vi "HVOF_DAQ.vi"() -> ()   [LabVIEW 2018]
uses:
  <vilib>/Enthought/Python Integration Toolkit/api/Console Visibility.ctl
  Global Variables.vi
  <vilib>/Enthought/Python Integration Toolkit/api/Unpack Double Array.vi
  <vilib>/Enthought/Python Integration Toolkit/Python Integration Toolkit.lvlib
  <vilib>/Analysis/NI_AALPro.lvlib
panel:
  in  "Clear":bool
  out "Delta T (water)":cluster{"X":dbl[], "Y":dbl[]}(graph)={"X"=[3626976328.9747047, 3626976329.2882648, 3626976329.537915, 3626976329.7875648, 3626976330.037215, 3626976330.2868648, 3626976330.536515, 3626976330.7861648, 3626976331.0358152, 3626976331.2844663, 3626976331.5341167, 3626976331.7837663, 3626976332.0334167, 3626976332.2830663, 3626976332.5327168, 3626976332.7823663, 3626976333.0320168, 3626976333.2816663, 3626976333.5313168, 3626976333.7809663, 3626976334.0306168, 3626976334.2802663, 3626976334.529917, 3626976334.7795663, 3626976335.029217, 3626976335.2788663, 3626976335.528517, 3626976335.7781663, 3626976336.027817, 3626976336.2774663, 3626976336.527117, 3626976336.7767663, 3626976337.026417, 3626976337.2760663, 3626976337.525717, 3626976337.7753663, 3626976338.025017, 3626976338.2746663, 3626976338.524317, 3626976338.7739663, 3626976339.023617, 3626976339.2732663, 3626976339.522917, 3626976339.7725663, 3626976340.022217, 3626976340.2718663, 3626976340.521517, 3626976340.7711663, 3626976341.020817, 3626976341.2704663, 3626976341.520117, 3626976341.7697663, 3626976342.019417, 3626976342.2690663, 3626976342.518717, 3626976342.7683663, 3626976343.018017, 3626976343.2676663, 3626976343.517317, 3626976343.7669663, 3626976344.016617, 3626976344.2662663, 3626976344.515917, 3626976344.7655663], "Y"=[0.016941995376026142, -0.0034307203438679323, -0.0012931560773346007, 0.010212766094994663, -0.0005542021339124403, -0.0017151365641332461, -0.0034042597751167136, 0.008075112661089179, 0.013062579982253908, -0.0017947808146345778, -0.00029020971273041596, -0.0277087398070357, -0.006043112142130269, 0.005251339553606016, 0.004908344665242481, -0.027207278935801327, -0.018287754627294817, 0.004037512931798659, 0.020003009075523437, 0.001715165849578426, 0.01781288109937762, 0.013511391362559522, -0.0009499695656778329, 0.0052251496198962855, -0.00475004623102393, 0.014091761079061627, 0.004354215535926187, -0.004143001067557606, 0.0008971989165296179, 0.0018736020359426675, 0.015543342306873598, 0.004459598401435727, -0.011294751416421889, 0.004275060252105334, -0.010450252501527757, -0.009605758581823665, 0.008154198125065903, 0.02092663018909846, -0.019185110047445164, -0.015358660324153561, -0.009447532053005858, -0.0005277680540594076, 0.009130734924596595, 0.01063513118945636, -0.00794342524870828, 0.008945990824315686, -0.008154211481919305, -0.00451269963069123, -0.005146015504564616, -0.0009762739930785358, -2.661033007456126e-05, 0.012745861399210412, -0.00044865324857923383, 0.005277504139456823, 0.006491598743970428, 0.004010972658196721, 0.0030610687129772884, -0.00451262343150205, 0.0032459063136975885, 0.0017681774285875917, -0.009763964236483957, -0.005330620501556638, -0.0016362406714414135, 0.027128009392132668]}
  in  "Clear":bool
  out "General XY Graph":cluster{"Y":dbl[], "Y":dbl[]}[](graph)=[{"Y"=[3626976328.9747047, 3626976329.2882648, 3626976329.537915, 3626976329.7875648, 3626976330.037215, 3626976330.2868648, 3626976330.536515, 3626976330.7861648, 3626976331.0358152, 3626976331.2844663, 3626976331.5341167, 3626976331.7837663, 3626976332.0334167, 3626976332.2830663, 3626976332.5327168, 3626976332.7823663, 3626976333.0320168, 3626976333.2816663, 3626976333.5313168, 3626976333.7809663, 3626976334.0306168, 3626976334.2802663, 3626976334.529917, 3626976334.7795663, 3626976335.029217, 3626976335.2788663, 3626976335.528517, 3626976335.7781663, 3626976336.027817, 3626976336.2774663, 3626976336.527117, 3626976336.7767663, 3626976337.026417, 3626976337.2760663, 3626976337.525717, 3626976337.7753663, 3626976338.025017, 3626976338.2746663, 3626976338.524317, 3626976338.7739663, 3626976339.023617, 3626976339.2732663, 3626976339.522917, 3626976339.7725663, 3626976340.022217, 3626976340.2718663, 3626976340.521517, 3626976340.7711663, 3626976341.020817, 3626976341.2704663, 3626976341.520117, 3626976341.7697663, 3626976342.019417, 3626976342.2690663, 3626976342.518717, 3626976342.7683663, 3626976343.018017, 3626976343.2676663, 3626976343.517317, 3626976343.7669663, 3626976344.016617, 3626976344.2662663, 3626976344.515917, 3626976344.7655663], "Y"=[5.746555713603573, 5.699783191946977, 5.753300065910536, 5.739767563942959, 5.784591234930852, 5.742044879207851, 5.834560760793132, 5.76162102278082, 5.800357252816253, 5.787463095545072, 5.768518652631912, 5.719227948241672, 5.777211861182645, 5.701929124682287, 5.720081940981363, 5.754241647220031, 5.742066778961799, 5.737599740402041, 5.763635566989369, 5.7283372027544965, 5.772876208570432, 5.765693913205542, 5.800291565032008, 5.781875977763636, 5.753190579724322, 5.778175339779396, 5.71064422770916, 5.718023598797108, 5.781963568315495, 5.761489637889099, 5.715155056662675, 5.780496451876758, 5.693892828585813, 5.765321656561875, 5.692338130932262, 5.795802625382005, 5.7746936776866535, 5.757570026557633, 5.7393515193935585, 5.791707843718633, 5.7383880394743105, 5.727811667047649, 5.7434244077143, 5.7520081297636265, 5.719030872886687, 5.690849111997867, 5.745679827512527, 5.7247898475659245, 5.755993424890152, 5.74605207668688, 5.724877438603042, 5.756212400427707, 5.7649494023393375, 5.757438645681126, 5.747935241465974, 5.7416069330134265, 5.73922013403042, 5.717016329940236, 5.716118537338039, 5.703067780408296, 5.767993119931336, 5.77541628947981, 5.725271587807375, 5.741278477750302]}]
  in  "Display":T1(ring)
  in  "Clear":bool caption="Reset"
  out "dM/dt (seed)":cluster{"X":dbl[], "Y":dbl[]}(graph)={"X"=[3626976329.2882648, 3626976329.537915, 3626976329.7875648, 3626976330.037215, 3626976330.2868648, 3626976330.536515, 3626976330.7861648, 3626976331.0358152, 3626976331.2844663, 3626976331.5341167, 3626976331.7837663, 3626976332.0334167, 3626976332.2830663, 3626976332.5327168, 3626976332.7823663, 3626976333.0320168, 3626976333.2816663, 3626976333.5313168, 3626976333.7809663, 3626976334.0306168, 3626976334.2802663, 3626976334.529917, 3626976334.7795663, 3626976335.029217, 3626976335.2788663, 3626976335.528517, 3626976335.7781663, 3626976336.027817, 3626976336.2774663, 3626976336.527117, 3626976336.7767663, 3626976337.026417, 3626976337.2760663, 3626976337.525717, 3626976337.7753663, 3626976338.025017, 3626976338.2746663, 3626976338.524317, 3626976338.7739663, 3626976339.023617, 3626976339.2732663, 3626976339.522917, 3626976339.7725663, 3626976340.022217, 3626976340.2718663, 3626976340.521517, 3626976340.7711663, 3626976341.020817, 3626976341.2704663, 3626976341.520117, 3626976341.7697663, 3626976342.019417, 3626976342.2690663, 3626976342.518717, 3626976342.7683663, 3626976343.018017, 3626976343.2676663, 3626976343.517317, 3626976343.7669663, 3626976344.016617, 3626976344.2662663, 3626976344.515917, 3626976344.7655663], "Y"=[-2.5294209395323057e-06, -4.259990571658549e-09, -1.2808149425667877e-11, 1.8085107227541341e-09, -5.379422771258245e-10, 1.5113616308576627e-10, 1.424266238208227e-09, 7.275029040386229e-10, -6.475231197382718e-10, 2.089720763854891e-09, -1.1450485775236743e-09, -1.3013079992401613e-09, 1.8981677703537083e-09, -1.0246515663609178e-11, -3.299379341274009e-09, -4.867097574581571e-11, -2.203001731242689e-09, 2.4950275467482267e-09, -2.3233983482318323e-09, 3.112380365943664e-09, -2.5769997091317265e-09, 3.885992600931171e-09, -1.869989848959745e-09, 2.1210295811829608e-09, -3.6118981658193606e-10, 3.775842497494251e-09, -4.651919934613945e-09, 1.869989846723482e-09, -5.338436771311457e-09, 5.8405162360633124e-09, -6.480923716412123e-09, 4.3522092517814356e-09, -4.651919953105369e-09, 5.520312497129659e-09, -5.507504346244076e-09, 7.257097584244414e-09, -2.23117966599756e-09, 2.664095121156259e-09, -3.276324674057799e-09, 3.873184442553429e-09, -2.5129589512684207e-09, 2.4822193848779224e-09, -5.153999395455975e-09, 1.6727443400957462e-09, -3.4351457380716585e-09, 1.4729372115131607e-09, -3.417214324594375e-09, 3.199475776996257e-09, -2.5949311204870922e-09, 6.2017060580144864e-09, -3.0790791737566973e-09, 3.809143702552645e-09, -2.279850629196931e-09, 4.449551178950508e-09, -4.444427917915515e-09, 4.380387168823738e-09, -5.940419799412757e-09, 4.252305674276681e-09, -2.748628906753415e-09, 4.201073105044614e-10, -2.3438913778313254e-09, 4.4572359918503736e-10, -1.7931409476573773e-09]}
  out "M (seed)":cluster{"X":dbl[], "Y":dbl[]}[](graph)=[{"X"=[3626976328.9747047, 3626976329.2882648, 3626976329.537915, 3626976329.7875648, 3626976330.037215, 3626976330.2868648, 3626976330.536515, 3626976330.7861648, 3626976331.0358152, 3626976331.2844663, 3626976331.5341167, 3626976331.7837663, 3626976332.0334167, 3626976332.2830663, 3626976332.5327168, 3626976332.7823663, 3626976333.0320168, 3626976333.2816663, 3626976333.5313168, 3626976333.7809663, 3626976334.0306168, 3626976334.2802663, 3626976334.529917, 3626976334.7795663, 3626976335.029217, 3626976335.2788663, 3626976335.528517, 3626976335.7781663, 3626976336.027817, 3626976336.2774663, 3626976336.527117, 3626976336.7767663, 3626976337.026417, 3626976337.2760663, 3626976337.525717, 3626976337.7753663, 3626976338.025017, 3626976338.2746663, 3626976338.524317, 3626976338.7739663, 3626976339.023617, 3626976339.2732663, 3626976339.522917, 3626976339.7725663, 3626976340.022217, 3626976340.2718663, 3626976340.521517, 3626976340.7711663, 3626976341.020817, 3626976341.2704663, 3626976341.520117, 3626976341.7697663, 3626976342.019417, 3626976342.2690663, 3626976342.518717, 3626976342.7683663, 3626976343.018017, 3626976343.2676663, 3626976343.517317, 3626976343.7669663, 3626976344.016617, 3626976344.2662663, 3626976344.515917, 3626976344.7655663], "Y"=[-9182.465313225688, -9174.149894063119, -9189.60077906248, -9189.647233917369, -9183.08780832068, -9185.038912230502, -9184.490744943321, -9179.324964999714, -9176.686329181648, -9179.034880214616, -9171.455512453122, -9175.608576548546, -9180.328389868973, -9173.443780282194, -9173.480944152043, -9185.447714949718, -9185.624243427048, -9193.614478576694, -9184.565072704409, -9192.991983534932, -9181.703453595828, -9191.050170561373, -9176.955767351936, -9183.738176284593, -9176.045252183509, -9177.355279101426, -9163.660387710675, -9180.532791235262, -9173.750382310716, -9193.112766156975, -9171.929351972754, -9195.435508934255, -9179.650148964256, -9196.52255255591, -9176.50050975583, -9196.476097695728, -9170.15477648218, -9178.247212334409, -9168.584602370387, -9180.467754435611, -9166.41980611353, -9175.5342487657, -9166.531297793439, -9185.224731641807, -9179.157727502385, -9191.616919808608, -9186.274611396524, -9198.668766890376, -9187.064343956321, -9196.476097726541, -9173.982656604929, -9185.150403907975, -9171.334729834483, -9179.603694118536, -9163.465277282094, -9179.585112171993, -9163.697551563655, -9185.243313608129, -9169.820301549724, -9179.789513553786, -9178.265794279574, -9186.767032843529, -9185.15040389643, -9191.654083682537]}]
  in  "Seed Channel":i32=2
  out "Data":T2={"Fuel Flow\n(L/hr)"=5.741278477750302, "O2 Flow\n(SLPM)"=0.0, "Phi"=-inf, "Q_water "=1.0866120412865794e-05, "Q_fuel"=-2.595149921295117e-10, "Delta T (C)"=0.027128009392132668, "Water Flow\n(L/min)"=5.741278477750302, "Chamber Pressure (PSI)"=14.690853351832978} {"Chamber Pressure (PSI)" scale=0.0..30.0; "Water Flow\n(L/min)" scale=6.0..40.0; "Delta T (C)" scale=0.0..100.0; "O2 Flow\n(SLPM)" scale=0.0..600.0; "Phi" scale=0.0..2.0; "Fuel Flow\n(L/hr)" scale=6.0..16.0; "Q_water" format="%#_3g"; "Q_fuel" format="%#_3g"}
  in  "stop":bool
  # "Torch"
  # "Fuel In"
  # "O2 In"
  # "Water In"
  # "Water Out"
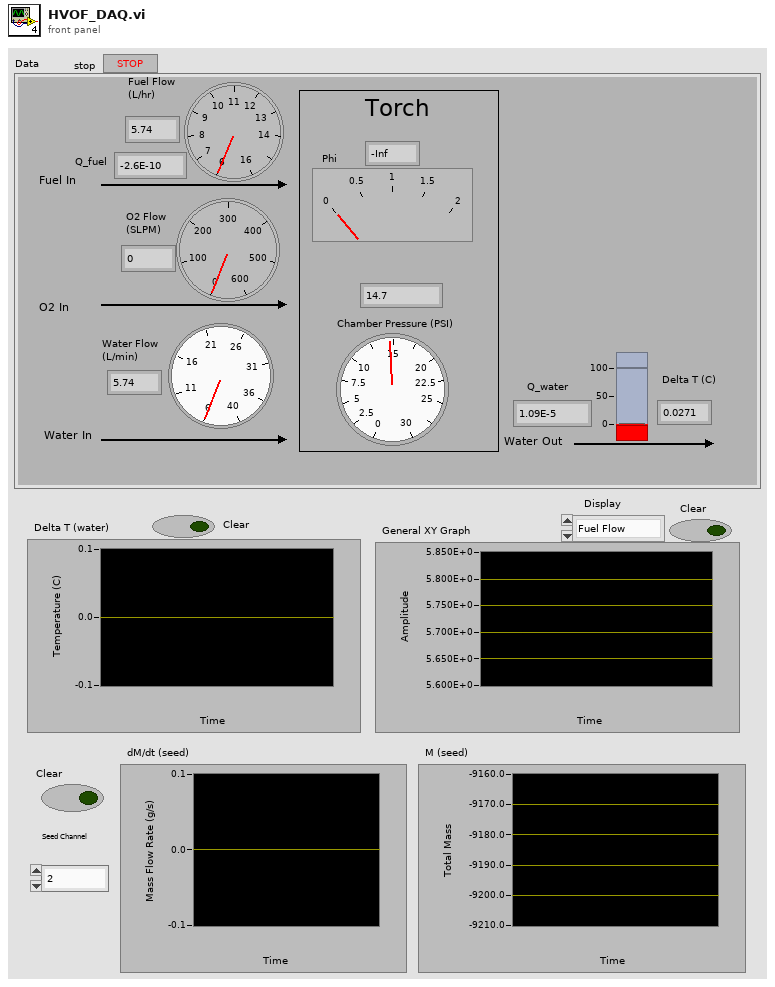
[diagram p1: front panel]
types:
  T1 = enum16{"Fuel Flow", "O2 Flow", "Phi", "Q_water", "Q_Fuel", "Delta T", "Water Flow", "Chamber Pressure"}
  T2 = cluster{"Fuel Flow\n(L/hr)":dbl, "O2 Flow\n(SLPM)":dbl, "Phi":dbl, "Q_water ":dbl, "Q_fuel":dbl, "Delta T (C)":dbl, "Water Flow\n(L/min)":dbl, "Chamber Pressure (PSI)":dbl}
  T3 = typedef "Python Integration Toolkit.lvlib/Console Visibility.ctl" = enum16{"Show Console", "Show Console While Running", "Hide Console"}
  T4 = typedef "Python Integration Toolkit.lvlib/Session ID.ctl" = u64
  T5 = typedef "Python Integration Toolkit.lvlib/Python Objects.ctl" = variant
  T6 = cluster{dbl, dbl, "Numeric":dbl, "Numeric":dbl, "Numeric":dbl, dbl, dbl, dbl}
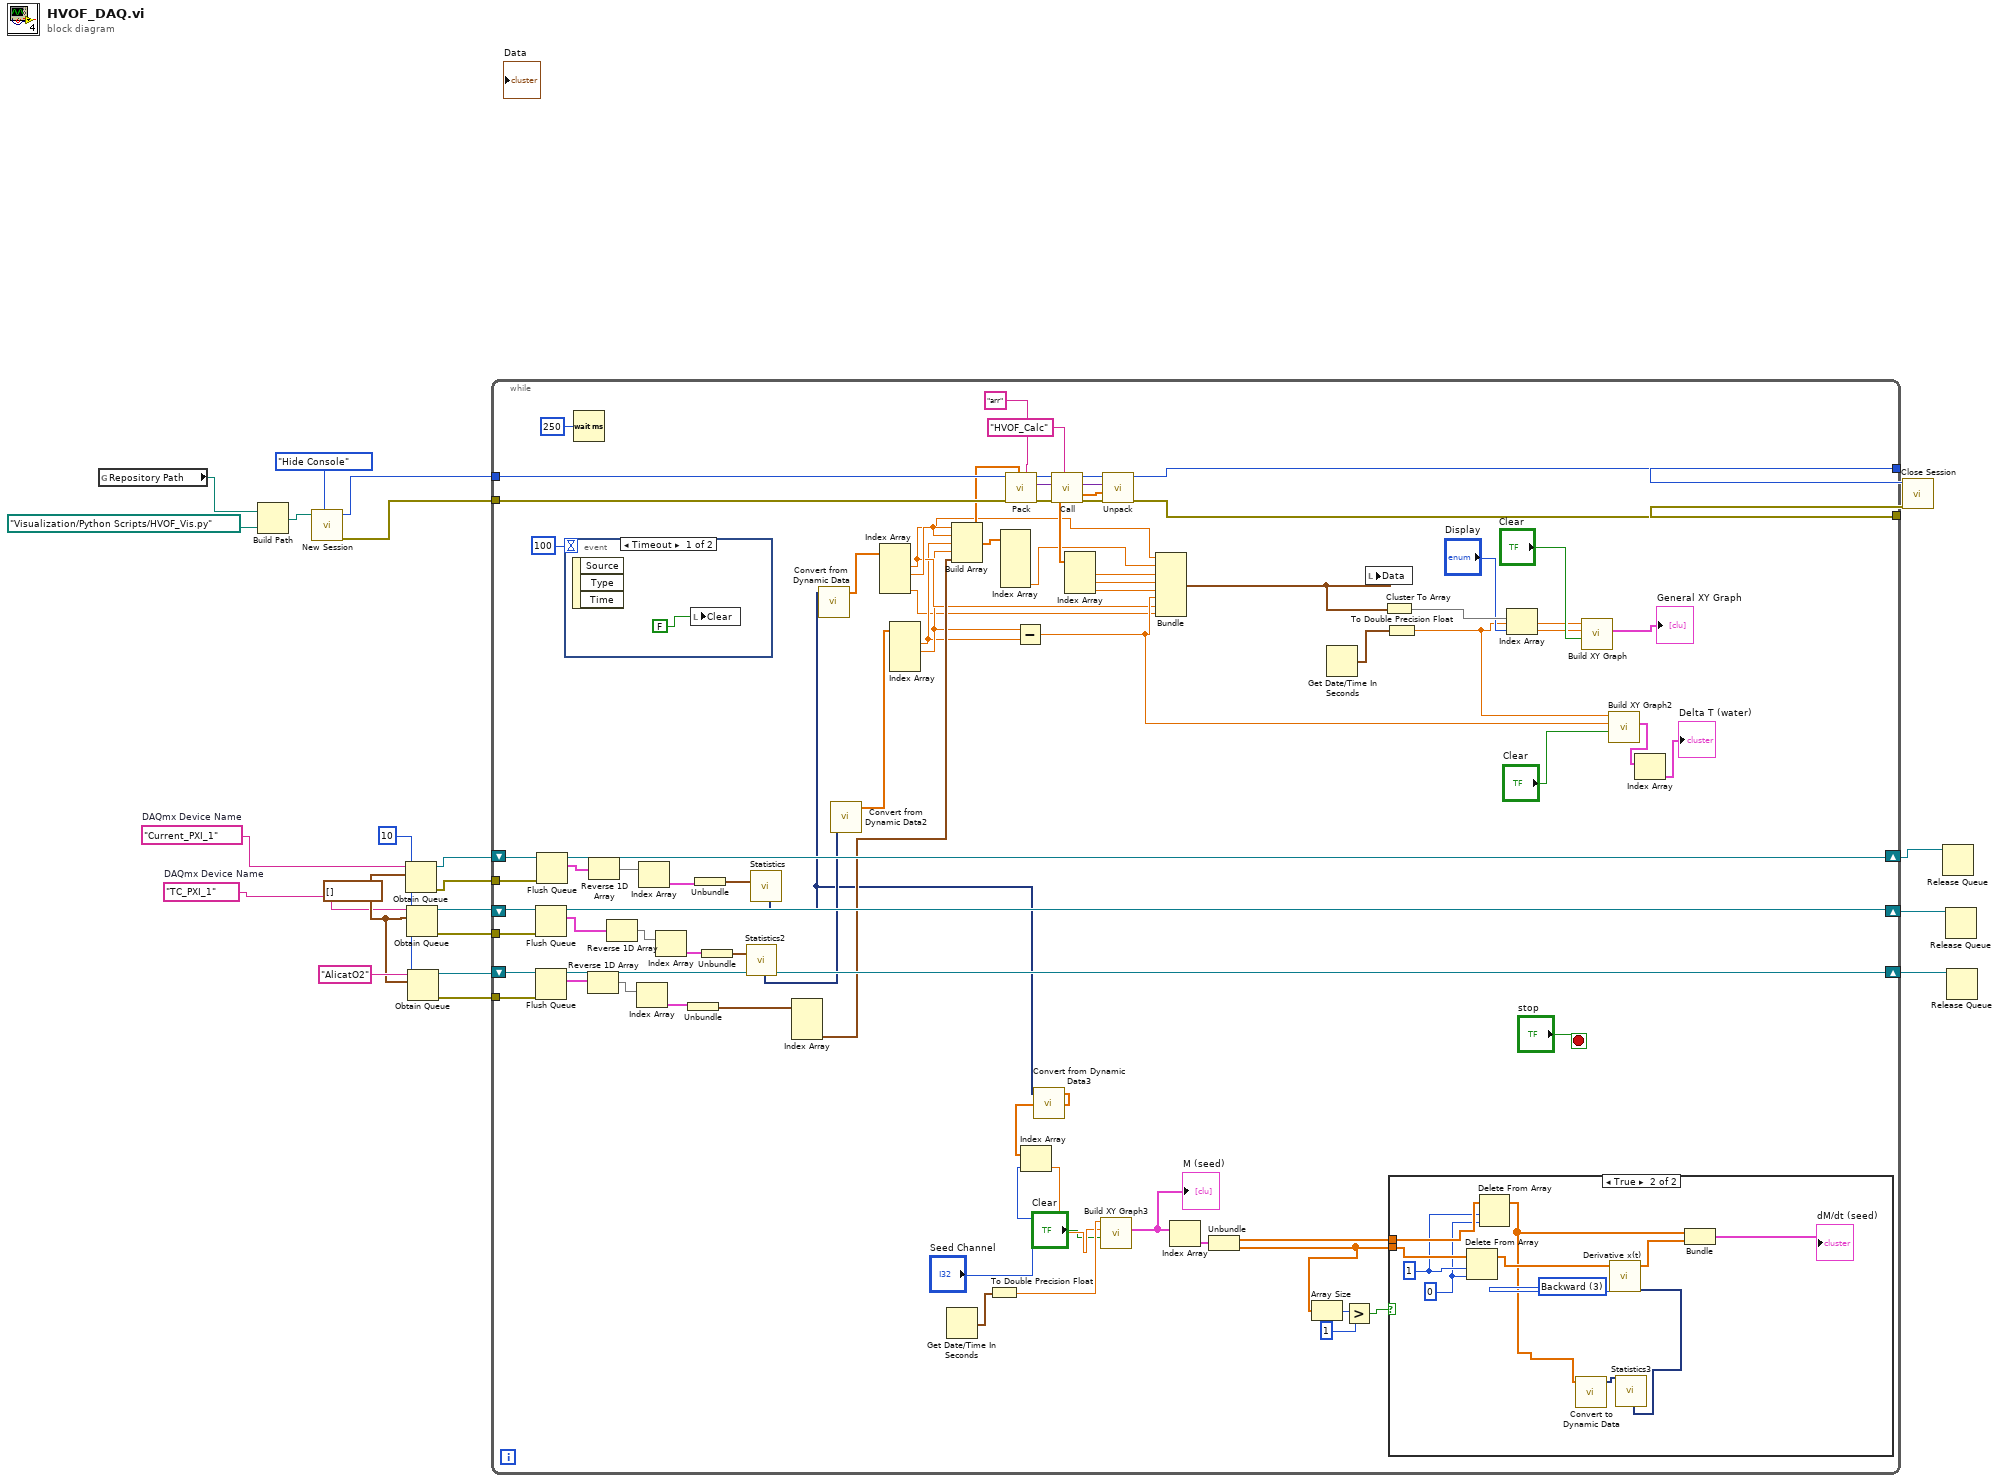
[diagram p0: block diagram]
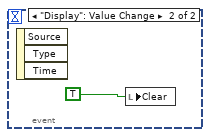
[diagram p3: hidden frame]
diagram:
  w1 = tag "TC_PXI_1"  # DAQmx Device Name
  w2 = tag "Current_PXI_1"  # DAQmx Device Name
  w17 = waveform(dbl)[] [] ("data")
  w6 = 10 ("max queue size (-1, unlimited)")
  n1 = global read "Global Variables.vi" "Repository Path"() -> (w11:path)
  n2 = Build Path(base path=w11, name or relative path=path "Visualization/Python Scripts/HVOF_Vis.py" ("vi path")) -> (appended path=w13:path)
  n3 = call <vilib>:"New Session.vi"("Console Visibility"=Console_Visibility."Hide Console", "Path to Python Module (.py File)"=w13) -> ("error out"=w9:errorcluster, "Session ID out"=w10:T4)  [unwired: 8 in]
  n4 = Obtain Queue(max queue size (-1, unlimited)=w6, name (unnamed)=w2, element data type=w17) -> (queue out=w22:refnum<queue>, error out=w20:errorcluster)  [unwired: 2 in, 1 out]
  n5 = Obtain Queue(max queue size (-1, unlimited)=w6, name (unnamed)=w1, element data type=w17) -> (queue out=w21:refnum<queue>, error out=w19:errorcluster)  [unwired: 2 in, 1 out]
  n6 = Obtain Queue(max queue size (-1, unlimited)=w6, name (unnamed)="AlicatO2", element data type=w17) -> (queue out=w16:refnum<queue>, error out=w15:errorcluster)  [unwired: 2 in, 1 out]
  n7 = while {
    shift-right: [w95] -> w4
    shift-left: w21 -> [w97]
    shift-right: [w96] -> w5
    shift-left: w22 -> [w98]
    tunnel: w20 -> [w92]
    tunnel: w19 -> [w91]
    shift-right: [w80] -> w3
    shift-left: w16 -> [w83]
    tunnel: w15 -> [w79]
    tunnel: w10 -> [w78]
    tunnel: w9 -> [w77]
    tunnel: [w68] -> w8
    tunnel: [w67] -> w7
    stop <- "stop" stop-if-true
    n8 = Flush Queue(queue=w97, error in (no error)=w91) -> (queue out=w95:refnum<queue>, remaining elements=w94:cluster{"data":waveform(dbl)[]}[])  [unwired: 1 out]
    n9 = Flush Queue(queue=w83, error in (no error)=w79) -> (queue out=w80:refnum<queue>, remaining elements=w81:cluster{"data":waveform(dbl)[]}[])  [unwired: 1 out]
    n10 = Flush Queue(queue=w98, error in (no error)=w92) -> (queue out=w96:refnum<queue>, remaining elements=w93:cluster{"data":waveform(dbl)[]}[])  [unwired: 1 out]
    n11 = event shown="[0] Timeout" {
      selector: _ -> [_ _]
      dyn-events: _ -> [_ _]
      timeout: 100 -> [_ _]
      event Timeout {
        n12 = event-data() -> ()  [unwired: 1 in, 3 out]
        n13 = local write "Clear"(FALSE) -> ()
      }
      event "Display": Value Change {
        n14 = event-data() -> ()  [unwired: 1 in, 3 out]
        n15 = local write "Clear"(TRUE) -> ()
      }
    }
    n16 = Wait (ms)(milliseconds to wait=u32 250) -> ()  [unwired: 1 out]
    n17 = Reverse 1D Array(array=w81) -> (reversed array=w82:cluster{"data":waveform(dbl)[]}[])
    n18 = Reverse 1D Array(array=w93) -> (reversed array=w90:cluster{"data":waveform(dbl)[]}[])
    n19 = Reverse 1D Array(array=w94) -> (reversed array=w89:cluster{"data":waveform(dbl)[]}[])
    n20 = Index Array(array=w82) -> (element=w63:cluster{"data":waveform(dbl)[]})  [unwired: 1 in]
    n21 = Index Array(array=w90) -> (element=w88:cluster{"data":waveform(dbl)[]})  [unwired: 1 in]
    n22 = Index Array(array=w89) -> (element=w87:cluster{"data":waveform(dbl)[]})  [unwired: 1 in]
    n23 = Unbundle(w63) -> ("data"=w62:waveform(dbl)[])
    n24 = Unbundle(w88) -> ("data"=w85:waveform(dbl)[])
    n25 = Unbundle(w87) -> ("data"=w84:waveform(dbl)[])
    n26 = call "Statistics2"("Signals"=w84) -> ("Arithmetic Mean"=w66:dynamicdata)  [unwired: 25 in, 1 out]
    n27 = call "Statistics"("Signals"=w85) -> ("Arithmetic Mean"=w32:dynamicdata)  [unwired: 25 in, 1 out]
    n28 = Index Array(array=w62) -> (element #3=w57:waveform(dbl))  [unwired: 3 in, 2 out]
    n29 = call "Convert from Dynamic Data"("Dynamic Data Type"=w32) -> ("Array"=w65:dbl[])  [unwired: 3 in]
    n30 = call "Convert from Dynamic Data2"("Dynamic Data Type"=w66) -> ("Array"=w64:dbl[])  [unwired: 3 in]
    n31 = Index Array(array=w65) -> (element #1=w41:dbl, element #2=w42:dbl, element #4=w23:dbl)  [unwired: 4 in, 1 out]
    n32 = Index Array(array=w64) -> (element #1=w39:dbl, element #2=w40:dbl)  [unwired: 4 in, 2 out]
    n33 = Get Date/Time In Seconds() -> (seconds since 1Jan1904=w38:timestamp)
    n34 = Build Array(w42, w41, w39, w40, w57) -> (w55:dbl[])
    n35 = To Double Precision Float(number=w38) -> (double precision float=w37:dbl)
    n36 = Index Array(array=w55) -> (element #5=w54:dbl)  [unwired: 5 in, 4 out]
    n37 = call <vilib>:"Pack.vi"("Keyword Name"="arr", "Argument"=w55, "error in (no error)"=w77, "Session ID"=w78) -> ("error out"=w76:errorcluster, "Python Object References Out"=w75:T5, "Session ID out"=w74:T4)  [unwired: 5 in]
    n38 = Subtract(x=w40, y=w39) -> (x-y=w47:dbl)
    n39 = call "Convert from Dynamic Data3"("Dynamic Data Type"=w32) -> ("Array"=w31:dbl[])  [unwired: 3 in]
    n40 = Index Array(array=w31, index="Seed Channel") -> (element=w30:dbl)
    n41 = call <vilib>:"Call.vi"("Function or Method Name"="HVOF_Calc" ("Python Code"), "error in (no error)"=w76, "Python Object References In"=w75, "Session ID"=w74) -> ("error out"=w71:errorcluster, "Python Object References Out"=w70:T5, "Session ID out"=w69:T4)  [unwired: 5 in]
    n42 = call "Build XY Graph3"("Reset"="Clear", "Y Input"=w30, "X Input"=w37) -> ("XY Graph"=w35:cluster{"X":dbl[], "Y":dbl[]}[])  [unwired: 7 in, 1 out]
    "M (seed)" <- w35
    n43 = call-poly <vilib>:"Unpack.vi"("error in (no error)"=w71, "Python Object References In"=w70, "Session ID"=w69) -> ("error out"=w67:errorcluster, "Value"=w61:dbl[], "Session ID out"=w68:T4)  [unwired: 5 in, 1 out]
    n44 = Index Array(array=w61) -> (element #1=w60:dbl, element #2=w59:dbl, element #3=w58:dbl)  [unwired: 3 in]
    n45 = Bundle(w41, w54, "Numeric"=w60, "Numeric"=w59, "Numeric"=w58, w47, w41, w23) -> (w56:T6)  [unwired: 1 in]
    n46 = Index Array(array=w35) -> (element=w36:cluster{"X":dbl[], "Y":dbl[]})  [unwired: 1 in]
    n47 = Unbundle(w36) -> ("X"=w34:dbl[], "Y"=w25:dbl[])
    n48 = Array Size(array=w25) -> (size(s)=w28:i32)
    n49 = Get Date/Time In Seconds() -> (seconds since 1Jan1904=w45:timestamp)
    n50 = Greater?(x=w28, y=1) -> (0:w26:bool)
    n51 = local write "Data"(w56) -> ()
    n52 = Cluster To Array(cluster=w56) -> (array=w51:dbl[])
    n53 = To Double Precision Float(number=w45) -> (double precision float=w46:dbl)
    n54 = case shown="True" w26 {
      tunnel: w25 -> [_ w104]
      tunnel: w34 -> [_ w105]
      frame False {
      }
      frame True {
        w101 = 0 ("index")
        w102 = 1 ("length")
        w110 = u16 3 items=["2nd Order Central", "4th Order Central", "Forward", "Backward"] ("method")
        n55 = Delete From Array(array=w104, length=w102, index=w101) -> (array with subset deleted=w103:dbl[])  [unwired: 1 out]
        n56 = Delete From Array(array=w105, length=w102, index=w101) -> (array with subset deleted=w100:dbl[])  [unwired: 1 out]
        n57 = call "Convert to Dynamic Data"("Array"=w100) -> ("Dynamic Data Type"=w107:dynamicdata)  [unwired: 3 in]
        n58 = call "Statistics3"("Signals"=w107) -> ("Arithmetic Mean"=w106:dynamicdata)  [unwired: 25 in, 1 out]
        n59 = call <vilib>:"Derivative x(t).vi"("method"=w110, "dt"=w106, "X"=w103) -> ("dX/dt"=w109:dbl[])  [unwired: 7 in, 1 out]
        n60 = Bundle("X"=w100, "dX/dt"=w109) -> (→"dM/dt (seed)":cluster{"X":dbl[], "dX/dt":dbl[]})  [unwired: 1 in]
      }
    }
    n61 = Index Array(array=w51, index="Display") -> (element=w49:dbl)
    n62 = call "Build XY Graph"("Reset"="Clear", "Y Input"=w49, "X Input"=w46) -> ("XY Graph"=→"General XY Graph":cluster{"X":dbl[], "Y":dbl[]}[])  [unwired: 7 in, 1 out]
    n63 = call "Build XY Graph2"("Reset"="Clear", "Y Input"=w47, "X Input"=w46) -> ("XY Graph"=w43:cluster{"X":dbl[], "Y":dbl[]}[])  [unwired: 7 in, 1 out]
    n64 = Index Array(array=w43) -> (element=→"Delta T (water)":cluster{"X":dbl[], "Y":dbl[]})  [unwired: 1 in]
  }
  n65 = call <vilib>:"Close Session.vi"("error in (no error)"=w7, "Session ID"=w8) -> ()  [unwired: 9 in, 1 out]
  n66 = Release Queue(queue=w5) -> ()  [unwired: 2 in, 3 out]
  n67 = Release Queue(queue=w4) -> ()  [unwired: 2 in, 3 out]
  n68 = Release Queue(queue=w3) -> ()  [unwired: 2 in, 3 out]
